vi "Load Previous Command.vi"(0 "Number of LBCBs":T1) -> ()   [LabVIEW 2009]
uses:
  Data Access Objects/Application/Number Of LBCBs.ctl
  Apps/App Parameters Actions.ctl
  Data Access Objects/Metadata/DAO Actions.ctl
  Data Access Objects/Metadata/LBCB Number.ctl
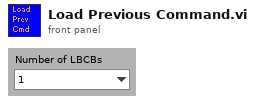
[diagram p1: front panel]
types:
  T1 = typedef "Number Of LBCBs.ctl" = enum16{"1", "2"}
  T2 = typedef "App Parameters Actions.ctl" = enum16{"Init", "Get", "Set"}
  T3 = typedef "App Parameters.ctl" = cluster{"Monitor Loop":T4, "Ramp Time":T4, "Log Loop":T4, "TCP to DAQ":T4, "Logging Directory":path, "Log File Size (MBytes)":i64, "Volt Logging Loop":T4, "2 LBCB Archiving Mode":bool}
  T4 = typedef "Timing Parameters.ctl" = cluster{"Interval":dbl, "Rate ":dbl}
  T5 = typedef "LBCB Number.ctl" = enum16{"LBCB1", "LBCB2"}
  T6 = enum16{"open", "replace", "create", "open or create", "replace or create", "replace or create with confirmation"}
  T7 = typedef "DAO Actions.ctl" = enum16{"Init", "Get", "Set"}
  T8 = typedef "Actuator Point.ctl" = cluster{"X1":dbl, "X2":dbl, "Y1":dbl, "Z1":dbl, "Z2":dbl, "Z3":dbl}
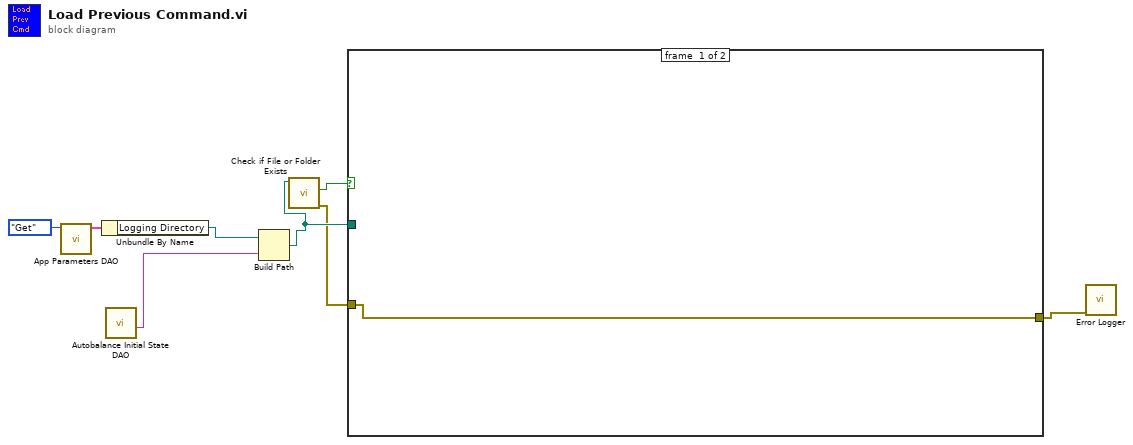
[diagram p0: block diagram]
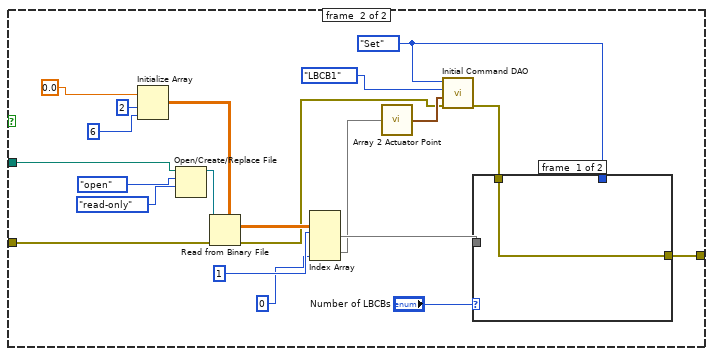
[diagram p2: hidden frame]
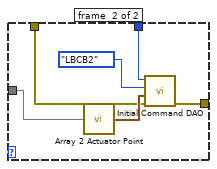
[diagram p3: hidden frame]
diagram:
  n1 = call "App Parameters DAO.vi"("Actions"=App_Parameters_Actions."Get" ("App Parameter Actions")) -> ("Application Timing and Logging Out"=w6:T3)  [unwired: 3 in, 7 out]
  n2 = Unbundle By Name(w6) -> ("Logging Directory"=w7:path)
  n3 = call "Autobalance Initial State DAO.vi"() -> ("autobalance\nfile"=w8:string)  [unwired: 2 in, 9 out]
  n4 = Build Path(base path=w7, name or relative path=w8) -> (appended path=w3:path)
  n5 = call <vilib>:"Check if File or Folder Exists.vi"("path"=w3) -> ("error out"=w1:errorcluster, "file or folder exists?"=w4:bool)  [unwired: 1 in, 8 out]
  n6 = case shown="True" w4 {
    tunnel: w3 -> [_ w23]
    tunnel: [w9 w16] -> w2
    tunnel: w1 -> [w9 w15]
    frame #0 {
    }
    frame #1 {
      w19 = DAO_Actions."Set" ("DAO Actions")
      n7 = Initialize Array(0.0, 2 ("dimension size"), 6 ("dimension size")) -> (w26:dbl[][])
      n8 = Open/Create/Replace File(file path (use dialog)=w23, operation (0:open)=T6."open", access (0:read/write)=enum16{"read/write", "read-only", "write-only"}."read-only") -> (refnum out=w30:refnum<file>)  [unwired: 1 in, 4 out]
      n9 = Read from Binary File(5:w26, 8:w15, 11:w30) -> (0:w18:errorcluster, 2:w25:dbl[][])  [unwired: 5 out]
      n10 = Index Array(array=w25, index (row) #1=1 ("length"), index (col) #2=0 ("length")) -> (element #1=w24:dbl[], element #2=w12:dbl[])  [unwired: 2 in]
      n11 = call "Array 2 Actuator Point.vi"("Array"=w12) -> ("Actuator Point"=w20:T8)
      n12 = call "Initial Command DAO.vi"("error in (no error)"=w18, "Command In"=w20, "LBCB Number"=LBCB_Number."LBCB1" ("Selected LBCB"), "DAO Actions"=w19) -> ("error out"=w17:errorcluster)  [unwired: 7 out]
      n13 = case shown="\"2\"" "Number of LBCBs" {
        tunnel: w24 -> [_ w37]
        tunnel: w19 -> [_ w35]
        tunnel: w17 -> [w31 w33]
        tunnel: [w31 w32] -> w16
        frame #0 {
        }
        frame #1 {
          n14 = call "Array 2 Actuator Point.vi"("Array"=w37) -> ("Actuator Point"=w36:T8)
          n15 = call "Initial Command DAO.vi"("error in (no error)"=w33, "Command In"=w36, "LBCB Number"=LBCB_Number."LBCB2" ("Selected LBCB"), "DAO Actions"=w35) -> ("error out"=w32:errorcluster)  [unwired: 7 out]
        }
      }
    }
  }
  n16 = call "Error Logger.vi"("error in (no error)"=w2) -> ()  [unwired: 1 in, 10 out]
